vi "Call_VI.vi"(2 "Target VI":string, 3 "File Path Control":path) -> (0 "String":string, 1 "Execution:State":T1(ring))   [LabVIEW 2015]
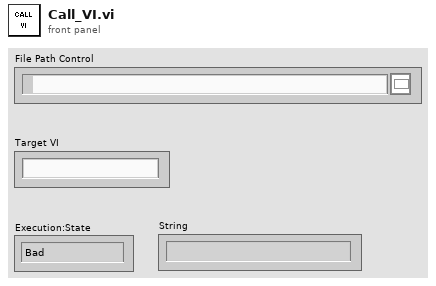
[diagram p1: front panel]
types:
  T1 = enum32{"Bad", "Idle", "Run top level", "Running"}
  T2 = enum32{"Invalid", "Standard", "Closed", "Hidden", "Minimized", "Maximized"}
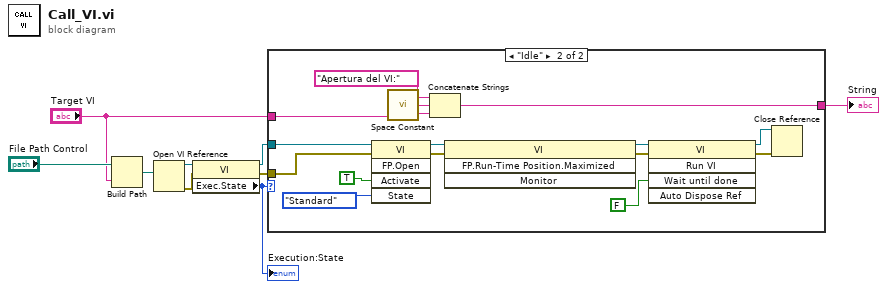
[diagram p0: block diagram]
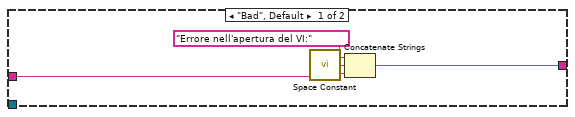
[diagram p2: hidden frame]
diagram:
  n1 = Build Path(base path="File Path Control", name or relative path="Target VI") -> (appended path=w8:path)
  n2 = Open VI Reference(vi path=w8) -> (vi reference=w4:refnum<vi>, error out=w5:errorcluster)  [unwired: 5 in]
  n3 = property class="VI"(reference=w4, error in=w5) -> (reference out=w6:refnum<vi>, error out=w7:errorcluster, "Exec.State"=w3:T1)
  "Execution:State" <- w3
  n4 = case shown="\"Idle\"" w3 {
    tunnel: w7 -> [_ w28]
    tunnel: w6 -> [_ w27]
    tunnel: "Target VI" -> [w11 w21]
    tunnel: [w10 w20] -> w1
    frame "Bad", Default {
      n5 = call <vilib>:"Space Constant.vi"() -> ("String"=w13:string)
      n6 = Concatenate Strings("Errore nell'apertura del VI:" ("String"), w13, w11) -> (w10:string)
    }
    frame "Idle" {
      n7 = invoke class="VI" method="FP.Open"(reference=w27, error in=w28, "Activate"=TRUE ("Activate?"), "State"=T2."Standard") -> (reference out=w19:refnum<vi>, error out=w17:errorcluster)  [unwired: 1 in, 3 out]
      n8 = call <vilib>:"Space Constant.vi"() -> ("String"=w22:string)
      n9 = Concatenate Strings("Apertura del VI:", w22, w21) -> (w20:string)
      n10 = invoke class="VI" method="FP.Run-Time Position.Maximized"(reference=w19, error in=w17) -> (reference out=w18:refnum<vi>, error out=w16:errorcluster)  [unwired: 2 in, 2 out]
      n11 = invoke class="VI" method="Run VI"(reference=w18, error in=w16, "Wait until done"=FALSE ("Wait Until Done")) -> (reference out=w25:refnum<vi>, error out=w26:errorcluster)  [unwired: 2 in, 3 out]
      n12 = Close Reference(reference=w25, error in (no error)=w26) -> ()  [unwired: 1 out]
    }
  }
  "String" <- w1
